vi "RS485 Write Rotork FPGA.vi"(10 "Valve SP":u8[](array[numeric])=[0, 0]) -> ()   [LabVIEW 2014]
uses:
  <vilib>/rvi/eio/common/nirviEmuTemplateMethod_errors.vi
  <vilib>/eio/EIOMethodNode/EIOMethodNode.xnode
panel:
  # "eg 0:    0   0\n500:     1   244\n1000:   3   232"
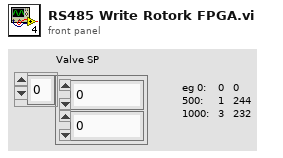
[diagram p1: front panel]
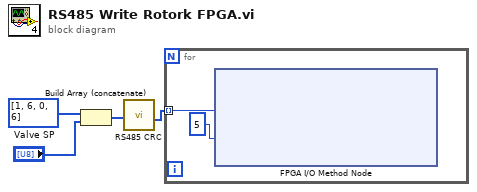
[diagram p0: block diagram]
diagram:
  n1 = Build Array (concatenate)(u8[] [1, 6, 0, 6] ("appended array"), "Valve SP") -> (w3:u8[])
  n2 = call "RS485 CRC.vi"("Data In"=w3) -> ("Data+CRC"=w1:u8[])  [unwired: 10 in]
  n3 = for {
    tunnel: w1 -> [w5] mode=indexing
    n4 = xnode "FPGA I/O Method Node"("Data"=w5, "Timeout (ms)"=5) -> ()  [unwired: 1 in, 2 out]
  }
